vi "ParseFileName.vi"(10 "Quantel File Name":string) -> (2 "File Parameters":T2)   [LabVIEW 2022 SP3]
panel:
  out "Cluster":T1
  out "length":i32
  out "remaining string":string
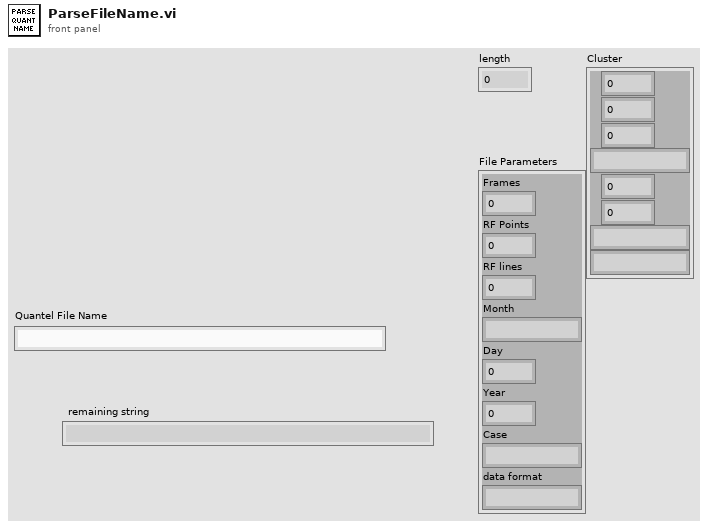
[diagram p1: front panel]
types:
  T1 = cluster{i32, i32, i32, string, i32, i32, string, string}
  T2 = cluster{"Frames":i32, "RF Points":i32, "RF lines":i32, "Month":string, "Day":i32, "Year":i32, "Case":string, "data format":string}
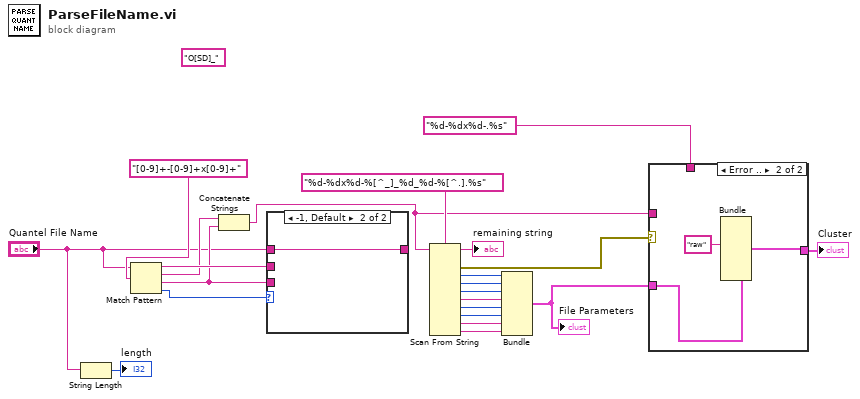
[diagram p0: block diagram]
diagram:
  (unwired) "O[SD]_" ("regular expression")
  n1 = String Length(string="Quantel File Name") -> (length=→"length":i32)
  n2 = Match Pattern(string="Quantel File Name", regular expression="[0-9]+-[0-9]+x[0-9]+" ("format string")) -> (before substring=w10:string, match substring=w9:string, after substring=w8:string, offset past match=w12:i32)  [unwired: 1 in]
  n3 = Concatenate Strings(w9, w8) -> (w3:string)
  n4 = case shown="-1, Default" w12 {
    tunnel: "Quantel File Name" -> [_ w24]
    tunnel: [w23 w24] -> _
    tunnel: w8 -> [w23 _]
    tunnel: w10 -> [_ _]
    frame 0 {
    }
    frame -1, Default {
    }
  }
  n5 = Scan From String(format string="%d-%dx%d-%[^_]_%d_%d-%[^.].%s", input string=w3) -> (remaining string=→"remaining string":string, error out=w5:errorcluster, output 1=w20:i32, output 2=w19:i32, output 3=w18:i32, output 4=w17:string, output 5=w16:i32, output 6=w15:i32, output 7=w14:string, output 8=w13:string)  [unwired: 10 in, 1 out]
  n6 = Bundle(w20, w19, w18, w17, w16, w15, w14, w13) -> (w2:T1)  [unwired: 1 in]
  "File Parameters" <- w2
  n7 = case shown="Error .." w5 {
    tunnel: "%d-%dx%d-.%s" ("format string") -> [_ _]
    tunnel: w3 -> [_ _]
    tunnel: w2 -> [w25 w28]
    tunnel: [w25 w27] -> w1
    frame No Error {
    }
    frame Error {
      n8 = Bundle(cluster=w28, "raw") -> (w27:T1)  [unwired: 7 in]
    }
  }
  "Cluster" <- w1
